vi "IsEmpty.vi"(8 "error in (no error)":errorcluster caption="错误输入（无错误）", 11 "Size输入":refnum<class "Size.lvclass">) -> (0 "error out":errorcluster caption="错误输出", 2 "Empty":bool, 3 "Size输出":refnum<class "Size.lvclass">)   [LabVIEW 2011, in "Size.lvclass"]
uses:
  Size.lvclass
  Size.lvclass/Size.ctl
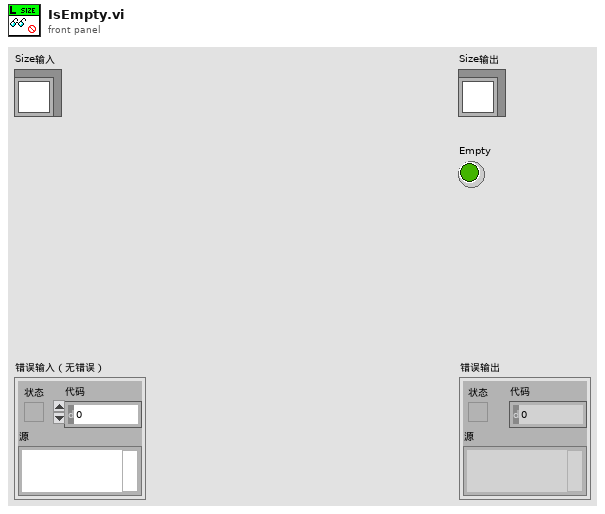
[diagram p1: front panel]
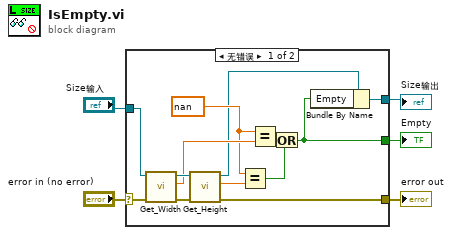
[diagram p0: block diagram]
diagram:
  n1 = case shown="无错误" "error in (no error)" {
    selector: "error in (no error)" -> [w16 w19]
    tunnel: [w6 w19] -> w4
    tunnel: [w7 w20] -> w2
    tunnel: "Size输入" -> [w18 w20]
    tunnel: [w8 _] -> w1
    frame No Error {
      w12 = nan ("y")
      n2 = call "Get_Width.vi"("error in (no error)"=w16, "Size输入"=w18) -> ("error out"=w15:errorcluster, "Width"=w14:dbl, "Size输出"=w17:refnum<class "Size.lvclass">)  [unwired: 7 in]
      n3 = call "Get_Height.vi"("error in (no error)"=w15, "Size输入"=w17) -> ("error out"=w6:errorcluster, "Height"=w13:dbl, "Size输出"=w9:refnum<class "Size.lvclass">)  [unwired: 7 in]
      n4 = Equal?(x=w12, y=w13) -> (x = y?=w10:bool)
      n5 = Equal?(x=w12, y=w14) -> (x = y?=w11:bool)
      n6 = Or(x=w11, y=w10) -> (x .or. y?=w8:bool)
      n7 = Bundle By Name(cluster=w9, "Empty"=w8) -> (w7:refnum<class "Size.lvclass">)
    }
    frame Error {
    }
  }
  "error out" <- w4
  "Size输出" <- w2
  "Empty" <- w1
